vi "UPTEST.vi"(6 "错误输入":errorcluster, 7 "Result":string[][](table), 8 "CODE_ID":string, 9 "DEVICE_ID":string) -> (0 "错误输出":errorcluster caption="错误输入")   [LabVIEW 2020]
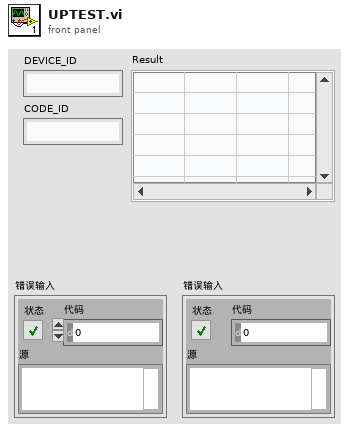
[diagram p1: front panel]
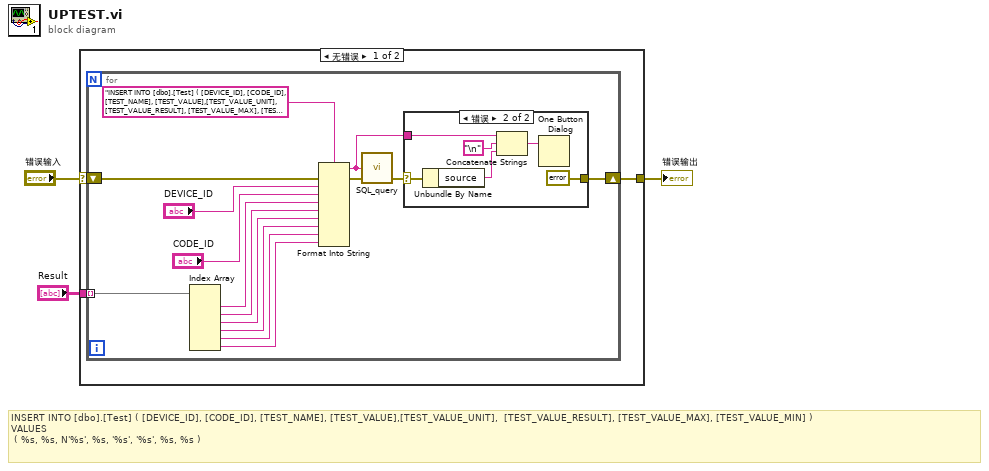
[diagram p0: block diagram]
diagram:
  # "INSERT INTO [dbo].[Test] ( [DEVICE_ID], [CODE_ID], [TEST_NAME], [TEST_VALUE],[TEST_VALUE_UNIT],  [TEST_VALUE_RESULT], [TEST_VALUE_MAX], [TEST_VALUE_MIN] )\nVALUES\n\t( %s, %s, N'%s', %s, '%s', '%s', %s, %s )"
  n1 = case shown="无错误" "错误输入" {
    selector: "错误输入" -> [w5 w29]
    tunnel: [w6 w29] -> w2
    tunnel: "Result" -> [w4 _]
    frame No Error {
      n2 = for {
        tunnel: w4 -> [w21] mode=indexing
        shift-right: [w10] -> w6
        shift-left: w5 -> [w14]
        n3 = Index Array(array=w21) -> (element #1=w20:string, element #2=w19:string, element #3=w18:string, element #4=w17:string, element #5=w16:string, element #6=w11:string)  [unwired: 6 in]
        n4 = Format Into String(format string="INSERT INTO [dbo].[Test] ( [DEVICE_ID], [CODE_ID], [TEST_NAME], [TEST_VALUE],[TEST_VALUE_UNIT],  [TEST_VALUE_RESULT], [TEST_VALUE_MAX], [TEST_VALUE_MIN] )\nVALUES\n\t( %s, %s, N'%s', %s, '%s', '%s', %s, %s )", error in=w14, "DEVICE_ID", "CODE_ID", w20, w19, w18, w17, w16, w11) -> (resulting string=w8:string, error out=w15:errorcluster)  [unwired: 1 in]
        n5 = call "SQL_query.vi"("error in (no error)"=w15, "SQL query"=w8) -> ("error out"=w9:errorcluster)  [unwired: 2 in, 1 out]
        n6 = case shown="错误" w9 {
          selector: w9 -> [w22 w27]
          tunnel: [w22 errorcluster {"status"=FALSE, "code"=0, "source"=""} ("error IO")] -> w10
          tunnel: w8 -> [_ w26]
          frame No Error {
          }
          frame Error {
            n7 = Unbundle By Name(w27) -> ("source"=w24:string)
            n8 = Concatenate Strings(w26, "\n", w24) -> (w23:string)
            n9 = One Button Dialog(message=w23) -> ()  [unwired: 1 in, 1 out]
          }
        }
      }
    }
    frame Error {
    }
  }
  "错误输出" <- w2
